vi "Stop Core.vi"(10 "final error code":i32, 11 "Tcp in":refnum<class "Tcp.lvclass">) -> (3 "Tcp out":refnum<class "Tcp.lvclass">)   [LabVIEW 2022 SP3, in "Tcp.lvlib" / "Tcp.lvclass"]
doc: "(<B>Filename</B>: Actor Framework.lvlib:Actor.lvclass:Stop Core.vi)\n\nDefines what the actor does before it stops. Use the <B>final error code</B> input to determine whether the actor shut down in response to an error.\n\nBy default, this method does nothing. A descendant class may override it to define behavior, such as shutting down any processes the actor initiated in its override of the Actor Core method."
uses:
  Tcp.lvclass
  C:/Users/jakub/repos/gh/sw4sys/lv-cli-framework/LoggingActor/Source/LoggingActor/LoggingActor/LoggingActor.lvclass
  Tcp.lvclass/Tcp.ctl
  LoggingActor/Source/LoggingActor/LoggingActor/LoggingActor.lvclass/LoggingActor.ctl
  LoggingActor/Source/LoggingActor/LoggingActor/Read Logger.vi
  Logger/Source/Logger/Logger.lvclass
  TcpSocket/Source/TcpSocket/TcpServer/TcpServer.lvclass
  LoggingActor/Source/LoggingActor/LoggingActor/LoggingActor.lvclass
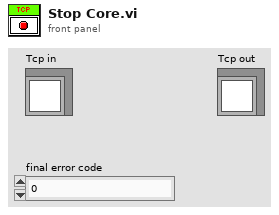
[diagram p1: front panel]
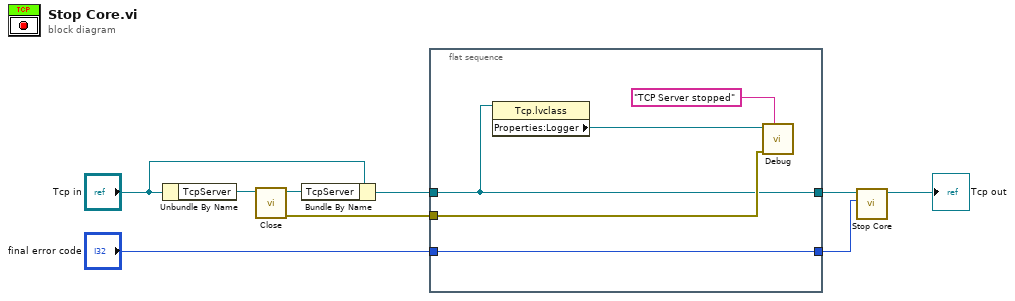
[diagram p0: block diagram]
diagram:
  n1 = Unbundle By Name("Tcp in") -> ("TcpServer"=w9:refnum<class "TcpServer.lvclass">)
  n2 = call-dynamic "Close.vi"("TcpSocket in"=w9) -> ("error out"=w7:errorcluster, "TcpSocket out"=w8:refnum<class "TcpServer.lvclass">)  [unwired: 9 in]
  n3 = Bundle By Name(cluster="Tcp in", "TcpServer"=w8) -> (w5:refnum<class "Tcp.lvclass">)
  n4 = flat-sequence {
    tunnel: w7 -> [w12]
    tunnel: w5 -> [w11]
    tunnel: "final error code" -> [w10]
    tunnel: [w11] -> w2
    tunnel: [w10] -> w1
    frame #0 {
      n5 = property class="Tcp.lvclass"(reference=w11) -> ("Properties:Logger"=w13:refnum<class "Logger.lvclass">)  [unwired: 1 in, 2 out]
      n6 = call-dynamic "Debug.vi"("Message"="TCP Server stopped", "error in (no error)"=w12, "Logger in"=w13) -> ()  [unwired: 7 in, 2 out]
    }
  }
  n7 = call-parent "Stop Core.vi"("final error code"=w1, "LoggingActor in"=w2) -> ("LoggingActor out"=→"Tcp out":refnum<class "Tcp.lvclass">)  [unwired: 9 in]
